vi "pp2_log_SpawnRLLogger.vi"(10 "file path in":path, 11 "queue in":refnum<queue>) -> ()   [LabVIEW 2013]
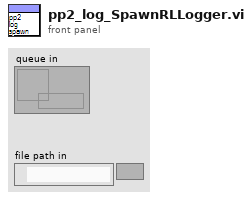
[diagram p1: front panel]
types:
  T1 = enum16{"open", "replace", "create", "open or create", "replace or create", "replace or create with confirmation"}
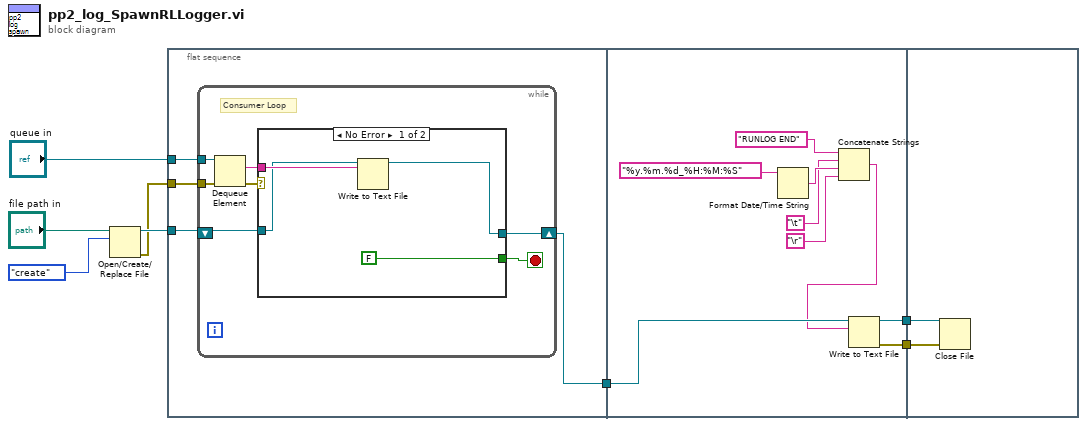
[diagram p0: block diagram]
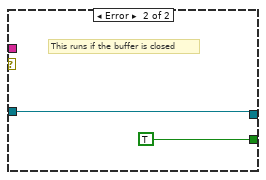
[diagram p2: hidden frame]
diagram:
  n1 = Open/Create/Replace File(file path (use dialog)="file path in", operation (0:open)=T1."create") -> (refnum out=w5:refnum<file>, error out=w2:errorcluster)  [unwired: 4 in, 1 out]
  n2 = flat-sequence {
    tunnel: "queue in" -> [w12]
    tunnel: w5 -> [w11]
    tunnel: [w9] -> w4
    tunnel: w2 -> [w10]
    tunnel: w4 -> [w34]
    tunnel: [w27] -> w3
    tunnel: [w26] -> w1
    tunnel: w3 -> [w36]
    tunnel: w1 -> [w35]
    frame #0 {
      n3 = while {
        tunnel: w12 -> [w17]
        tunnel: w10 -> [w15]
        shift-right: [w13] -> w9
        shift-left: w11 -> [w16]
        stop <- w19 stop-if-true
        # "Consumer Loop"
        n4 = Dequeue Element(queue=w17, error in (no error)=w15) -> (element=w18:string, error out=w14:errorcluster)  [unwired: 1 in, 2 out]
        n5 = case shown="No Error" w14 {
          tunnel: [FALSE TRUE] -> w19
          tunnel: w18 -> [w22 _]
          tunnel: w16 -> [w21 w24]
          tunnel: [w20 w24] -> w13
          frame No Error {
            n6 = Write to Text File(file (use dialog)=w21, text=w22) -> (refnum out=w20:refnum<file>)  [unwired: 2 in, 2 out]
          }
          frame Error {
            # "This runs if the buffer is closed"
          }
        }
      }
    }
    frame #1 {
      n7 = Format Date/Time String(time format string (%c)="%y.%m.%d_%H:%M:%S" ("pattern (all files)")) -> (date/time string=w33:string)  [unwired: 2 in]
      n8 = Concatenate Strings("RUNLOG END" ("string"), "\t", w33, "\r") -> (w28:string)
      n9 = Write to Text File(file (use dialog)=w34, text=w28) -> (refnum out=w27:refnum<file>, error out=w26:errorcluster)  [unwired: 2 in, 1 out]
    }
    frame #2 {
      n10 = Close File(refnum=w36, error in=w35) -> ()  [unwired: 2 out]
    }
  }
